vi "DataCluster.vi"(8 "error in (no error)":errorcluster) -> (0 "error out":errorcluster, 3 "Data Cluster":T1)   [LabVIEW 2013, in "UserConsole.lvlib"]
uses:
  UserConsole.lvlib
  PrivateControls/DataCluster.ctl
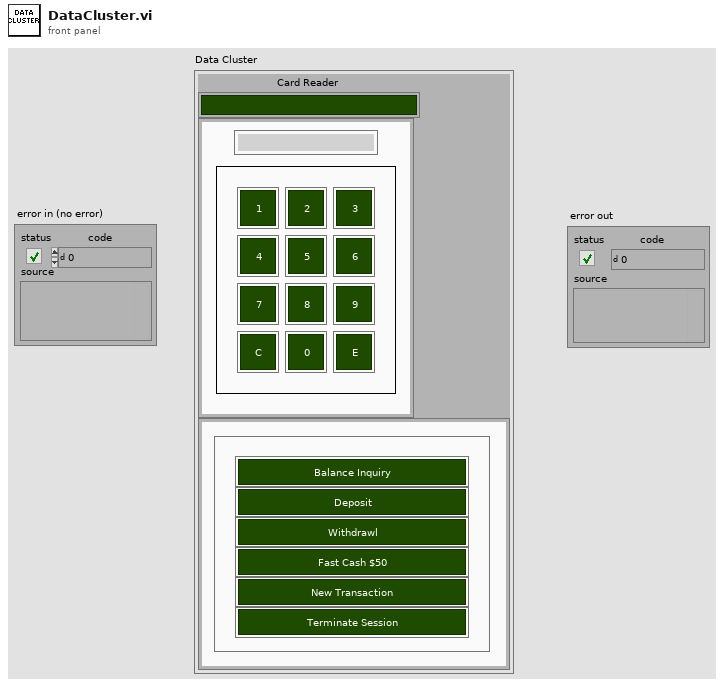
[diagram p1: front panel]
types:
  T1 = typedef "UserConsole.lvlib/DataCluster.ctl" = cluster{"Card Reader":bool, "Keypad":cluster{"Key":bool, "Key 2":bool, "Key 3":bool, "Key 4":bool, "Key 5":bool, "Key 6":bool, "Key 7":bool, "Key 8":bool, "Key 9":bool, "Key 10":bool, "Key 11":bool, "Key 12":bool, "Knumber":string}, "Transactions":cluster{"xaction":bool, "xaction 2":bool, "xaction 3":bool, "xaction 4":bool, "xaction 5":bool, "xaction 6":bool}}
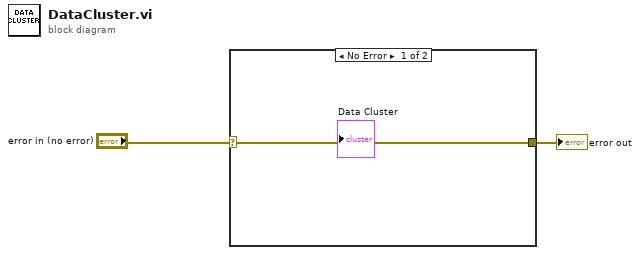
[diagram p0: block diagram]
diagram:
  n1 = case shown="No Error" "error in (no error)" {
    selector: "error in (no error)" -> [w3 w4]
    tunnel: [w3 w4] -> w1
    frame No Error {
    }
    frame Error {
    }
  }
  "error out" <- w1
